vi "odometry.vi"(1 "reset":bool, 2 "distance between sides of wheels":dbl, 3 "encoders in":dbl[](array[numeric]), 4 "state in":dbl[](array[numeric])) -> (0 "state out":dbl[](array[numeric]))   [LabVIEW 2016]
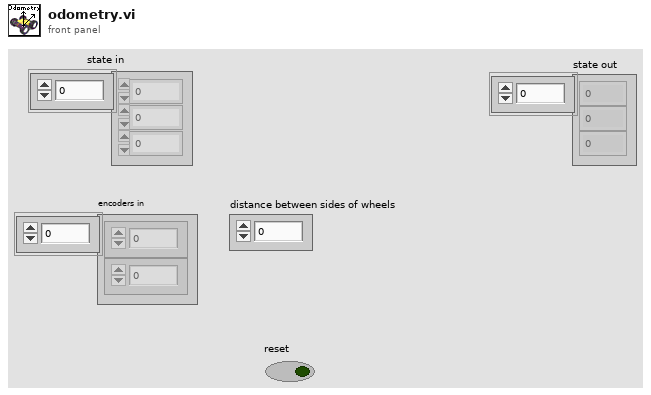
[diagram p1: front panel]
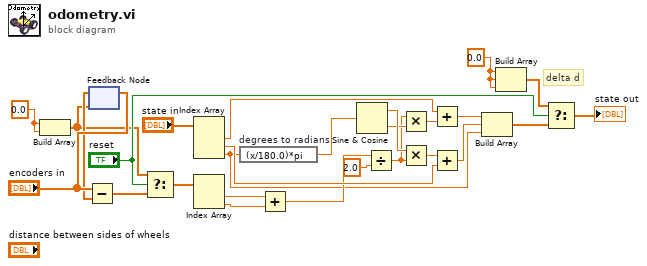
[diagram p0: block diagram]
diagram:
  w8 = 0.0 ("element")
  w15 = 0.0 ("element")
  # "delta d"
  n1 = Build Array(w15, w15) -> (w9:dbl[])
  n2 = feedback-in #1("encoders in") -> ()
  n3 = feedback #1(w9) -> (w13:dbl[])
  n4 = Subtract(x="encoders in", y=w13) -> (x-y=w6:dbl[])
  n5 = Select(t=w9, s="reset", f=w6) -> (s? t:f=w5:dbl[])
  n6 = Index Array(array="state in") -> (element #1=w20:dbl, element #2=w19:dbl, element #3=w1:dbl)  [unwired: 3 in]
  n7 = Index Array(array=w5) -> (element #1=w2:dbl, element #2=w16:dbl)  [unwired: 2 in]
  n8 = expression code="(x/180.0)*pi" "degrees to radians"(w1) -> (w27:dbl)
  n9 = Add(x=w2, y=w16) -> (x+y=w4:dbl)
  n10 = Sine & Cosine(0:w27) -> (1:w25:dbl, 2:w24:dbl)
  n11 = Divide(x=w4, y=2.0) -> (x/y=w23:dbl)
  n12 = Multiply(x=w23, y=w24) -> (x*y=w3:dbl)
  n13 = Multiply(x=w25, y=w23) -> (x*y=w22:dbl)
  n14 = Add(x=w20, y=w3) -> (x+y=w18:dbl)
  n15 = Add(x=w22, y=w19) -> (x+y=w17:dbl)
  n16 = Build Array(w18, w17, w1) -> (w12:dbl[])
  n17 = Build Array(w8, w8, w8) -> (w7:dbl[])
  n18 = Select(t=w7, s="reset", f=w12) -> (s? t:f=→"state out":dbl[])
